vi "_Init for constructor.vi"(8 "error in (no error)":errorcluster, 10 "Parameters":T1, 11 "DualScreen in":refnum<class "DualScreen.lvclass">) -> (0 "error out":errorcluster, 3 "DualScreen out":refnum<class "DualScreen.lvclass">)   [LabVIEW 2020, in "DualScreen.lvlib" / "DualScreen.lvclass"]
uses:
  DualScreen.lvclass
  DualScreenParam.ctl
  support/UI_Actor.lvlibp/UI_Actor/UI_Actor.lvclass
  DualScreen.lvclass/DualScreen.ctl
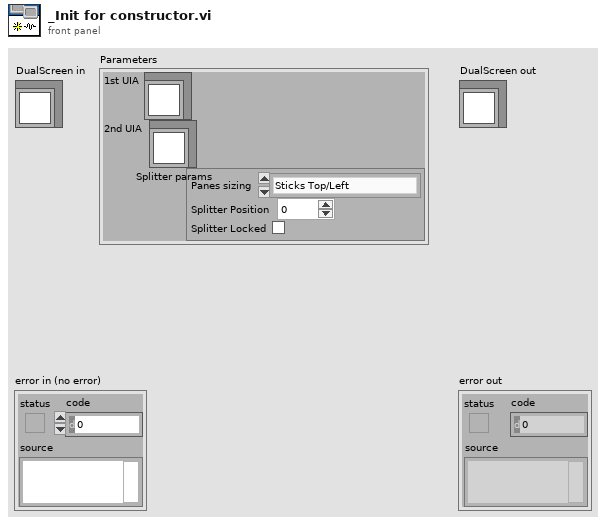
[diagram p1: front panel]
types:
  T1 = typedef "DualScreen.lvlib/DualScreen.lvclass/DualScreenParam.ctl" = cluster{"1st UIA":refnum<class "UI_Actor.lvclass">, "2nd UIA":refnum<class "UI_Actor.lvclass">, "Splitter params":cluster{"Panes sizing":enum16{"Sticks Top/Left", "Sticks Bottom/Right", "Proportional"}, "Splitter Position":i32, "Splitter Locked":bool}}
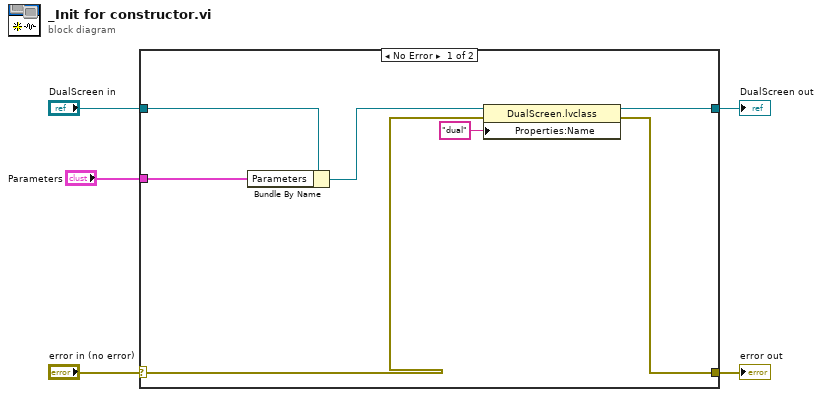
[diagram p0: block diagram]
diagram:
  n1 = case shown="No Error" "error in (no error)" {
    selector: "error in (no error)" -> [w7 w14]
    tunnel: [w6 w14] -> w4
    tunnel: [w8 w13] -> w2
    tunnel: "DualScreen in" -> [w12 w13]
    tunnel: "Parameters" -> [w11 _]
    frame No Error {
      n2 = Bundle By Name(cluster=w12, "Parameters"=w11) -> (w9:refnum<class "DualScreen.lvclass">)
      n3 = property class="DualScreen.lvclass"(reference=w9, error in=w7, "Properties:Name"="dual" ("Name")) -> (reference out=w8:refnum<class "DualScreen.lvclass">, error out=w6:errorcluster)
    }
    frame Error {
    }
  }
  "error out" <- w4
  "DualScreen out" <- w2
